vi "VolumeFlowCalculator_1.vi"() -> ()   [LabVIEW 2014]
panel:
  out "?":dbl(slide) scale=0.0..2000.0
  out "?":dbl(slide) scale=0.0..2000.0
  out "?":dbl
  out "?":dbl
  out "?":dbl
  out "?":dbl
  in  "?":dbl(slide) scale=0.0..1000.0
  in  "Gas Constant":dbl(slide) scale=0.0..400.0
  in  "Coefficient of Outflow C":dbl(slide) scale=0.0..2.0
  in  "Density of Liquid":dbl(slide) scale=0.0..2.0
  in  "Pressure in Position 2":dbl(slide) scale=0.0..200000.0
  in  "Pressure in Position 1":dbl(slide) scale=0.0..200000.0
  in  "Diameter of Tube in Position 2":dbl(slide) scale=0.0..300.0
  in  "Diameter of Tube in Position 1":dbl(slide) scale=0.0..300.0
  in  "Gas/Liquid":bool
  # "ECE 4342: Lab 6 - Volumetric Flow Calculator - Spring 2015 - Abhishek Barla (ID: 900559822)"
  # "Inputs"
  # "Outputs"
  # "Velocity in Position 1"
  # "Velocity in Position 2"
  # "Liquid"
  # "mm"
  # "Gas"
  # "m/s"
  # "m/s"
  # "Volumetric Flow"
  # "l/s"
  # "Mass Flow"
  # "g/s"
  # "mm"
  # "Pa"
  # "Temperature"
  # "Pa"
  # "K"
  # "Kg/m^3"
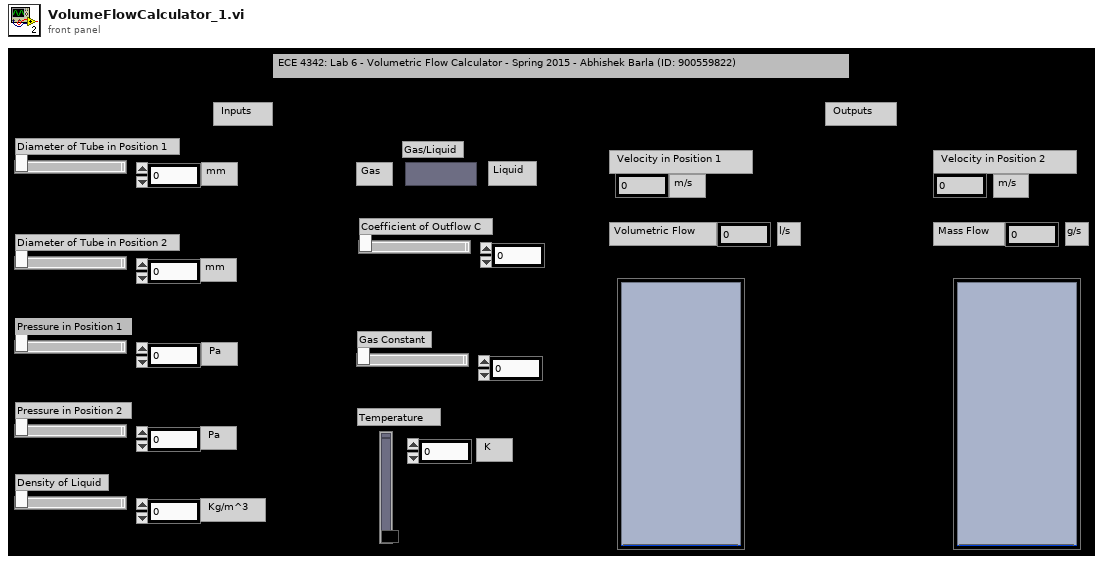
[diagram p1: front panel]
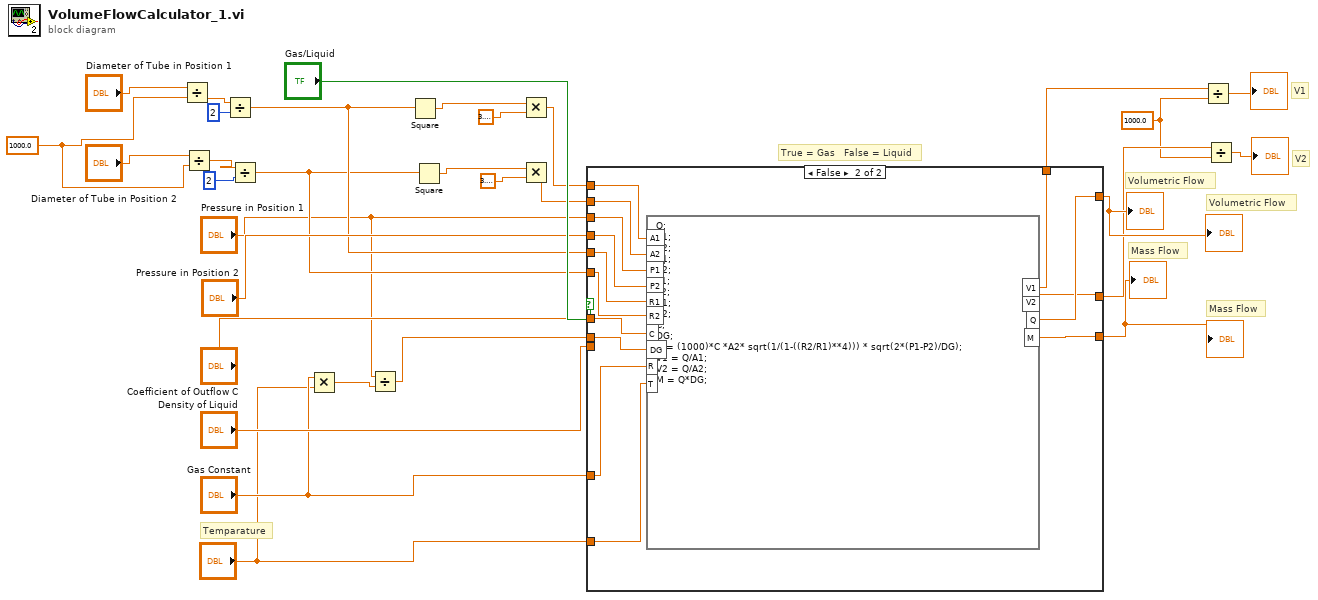
[diagram p0: block diagram]
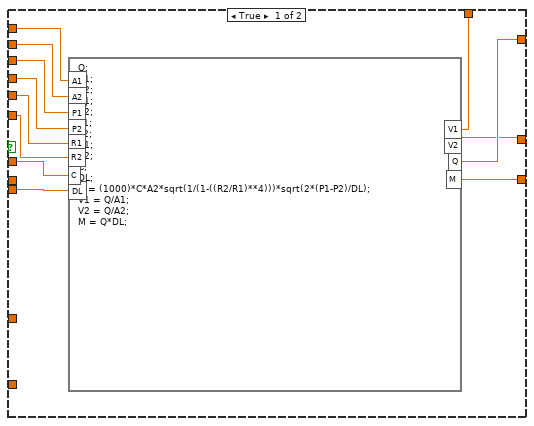
[diagram p2: hidden frame]
diagram:
  w1 = 1000.0
  w15 = 1000.0
  # "Mass Flow"
  # "Volumetric Flow"
  # "True = Gas   False = Liquid"
  # "Volumetric Flow"
  # "V1"
  # "Mass Flow"
  # "V2"
  # "Temparature"
  n1 = Divide(x="Diameter of Tube in Position 1", y=w15) -> (x/y=w13:dbl)
  n2 = Divide(x="Diameter of Tube in Position 2", y=w15) -> (x/y=w14:dbl)
  n3 = Divide(x=w13, y=2) -> (x/y=w22:dbl)
  n4 = Divide(x=w14, y=2) -> (x/y=w21:dbl)
  n5 = Multiply(x="Gas Constant", y="?") -> (x*y=w7:dbl)
  n6 = Divide(x="Pressure in Position 1", y=w7) -> (x/y=w6:dbl)
  n7 = Square(x=w22) -> (x^2=w28:dbl)
  n8 = Square(x=w21) -> (x^2=w27:dbl)
  n9 = Multiply(x=w28, y=3.141592653589793) -> (x*y=w25:dbl)
  n10 = Multiply(x=w27, y=3.141592653589793) -> (x*y=w24:dbl)
  n11 = case shown="False" "Gas/Liquid" {
    tunnel: w25 -> [w43 w57]
    tunnel: w24 -> [w42 w56]
    tunnel: "Pressure in Position 1" -> [w41 w55]
    tunnel: "Pressure in Position 2" -> [w40 w54]
    tunnel: w22 -> [w39 w53]
    tunnel: w21 -> [w38 w52]
    tunnel: [w37 w51] -> w19
    tunnel: "Density of Liquid" -> [w36 _]
    tunnel: "Coefficient of Outflow C" -> [w35 w50]
    tunnel: [w34 w49] -> w5
    tunnel: [w33 w48] -> w4
    tunnel: [w32 w47] -> w18
    tunnel: "Gas Constant" -> [_ w46]
    tunnel: "?" -> [_ w45]
    tunnel: w6 -> [_ w44]
    frame True {
      n12 = formula code="Q;\nA1;\nA2;\nV1;\nV2;\nP1;\nP2;\nR1;\nR2;\nC;\nDL;\nQ = (1000)*C*A2*sqrt(1/(1-((R2/R1)**4)))*sqrt(2*(P1-P2)/DL);\nV1 = Q/A1;\nV2 = Q/A2;\nM = Q*DL;"("A1"=w43, "A2"=w42, "P1"=w41, "P2"=w40, "R1"=w39, "R2"=w38, "DL"=w36, "C"=w35) -> ("Q"=w37:dbl, "V2"=w33:dbl, "V1"=w34:dbl, "M"=w32:dbl)
    }
    frame False {
      n13 = formula code="Q;\nA1;\nA2;\nV1;\nV2;\nP1;\nP2;\nR1;\nR2;\nC;\nDG; \nQ = (1000)*C *A2* sqrt(1/(1-((R2/R1)**4))) * sqrt(2*(P1-P2)/DG);\nV1 = Q/A1;\nV2 = Q/A2;\nM = Q*DG;"("A1"=w57, "A2"=w56, "P1"=w55, "P2"=w54, "R1"=w53, "R2"=w52, "C"=w50, "R"=w46, "T"=w45, "DG"=w44) -> ("Q"=w51:dbl, "V2"=w48:dbl, "V1"=w49:dbl, "M"=w47:dbl)
    }
  }
  "?" <- w19
  "?" <- w18
  "?" <- w19
  "?" <- w18
  n14 = Divide(x=w5, y=w1) -> (x/y=→"?":dbl)
  n15 = Divide(x=w4, y=w1) -> (x/y=→"?":dbl)
